vi "AOTF_Configuration.vi"(5 "error out":errorcluster) -> (19 "error out 2":errorcluster)   [LabVIEW 2011]
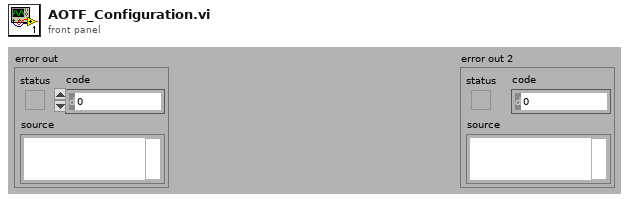
[diagram p1: front panel]
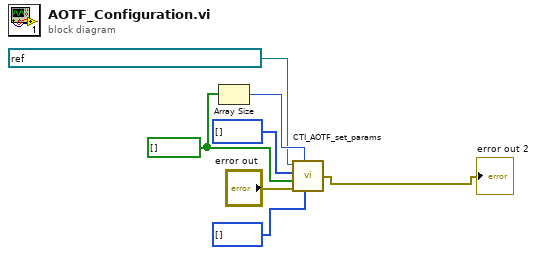
[diagram p0: block diagram]
diagram:
  w2 = bool[] [] ("LaserAOTFOnOff")
  n1 = Array Size(array=w2) -> (size(s)=w7:i32)
  n2 = call "CTI_AOTF_set_params.vi"("frequency"=i32[] [] ("WavelengthAOTF"), "Numeric"=w7, "error IO"="error out", "Array"=w2, "amplitude"=i16[] [] ("PowerChannelAotf"), "CTI AOTF-Controller"=refnum<visa-resource-name> "USB0::0x16C7::0x0001::NI-VISA-20001::RAW" ("VISA resource name 2")) -> ("error out"=→"error out 2":errorcluster)
